vi "ludlRead.vi"() -> (1 "X":i32, 2 "Y":i32, 3 "string":string)   [LabVIEW 2017]
uses:
  globalDevices.vi
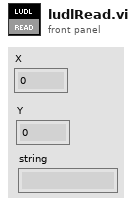
[diagram p1: front panel]
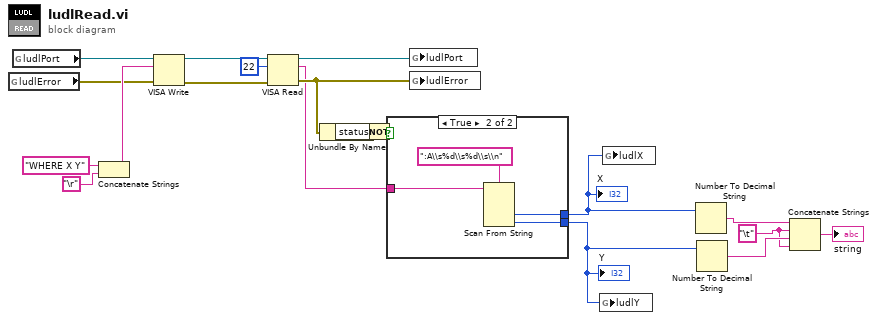
[diagram p0: block diagram]
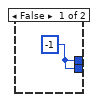
[diagram p2: hidden frame]
diagram:
  w5 = "\t" ("string")
  n1 = global read "globalDevices.vi" "ludlError"() -> (w16:errorcluster)
  n2 = global read "globalDevices.vi" "ludlPort"() -> (w15:refnum<visa-resource-name>)
  n3 = Concatenate Strings("WHERE X Y" ("string"), "\r") -> (w17:string)
  n4 = VISA Write(VISA resource name=w15, write buffer=w17, error in (no error)=w16) -> (VISA resource name out=w14:refnum<visa-resource-name>, error out=w13:errorcluster)  [unwired: 1 out]
  n5 = VISA Read(VISA resource name=w14, byte count=u32 22, error in (no error)=w13) -> (VISA resource name out=w11:refnum<visa-resource-name>, read buffer=w8:string, error out=w10:errorcluster)  [unwired: 1 out]
  n6 = Unbundle By Name(w10) -> ("status"=w9:bool)
  n7 = Not(x=w9) -> (.not. x?=w3:bool)
  n8 = case shown="True" w3 {
    tunnel: w8 -> [_ w23]
    tunnel: [w20 w22] -> w2
    tunnel: [w20 w21] -> w1
    frame False {
      w20 = -1
    }
    frame True {
      n9 = Scan From String(format string=":A\\s%d\\s%d\\s\\n", input string=w23) -> (output 1=w22:i32, output 2=w21:i32)  [unwired: 4 in, 3 out]
    }
  }
  "X" <- w2
  "Y" <- w1
  n10 = global write "globalDevices.vi" "ludlPort"(w11) -> ()
  n11 = global write "globalDevices.vi" "ludlError"(w10) -> ()
  n12 = global write "globalDevices.vi" "ludlY"(w1) -> ()
  n13 = global write "globalDevices.vi" "ludlX"(w2) -> ()
  n14 = Number To Decimal String(number=w2) -> (decimal integer string=w7:string)  [unwired: 1 in]
  n15 = Number To Decimal String(number=w1) -> (decimal integer string=w6:string)  [unwired: 1 in]
  n16 = Concatenate Strings(w7, w5, w6, w5) -> (→"string":string)
